vi "Impedance_Single_Meas.vi"(11 "Test Params Cluster":T1={"Test Freq. (Hz)"=1702.3933752476319, "Output Signal Amplitude\nVolts Pk"=0.1, "Sampling Time (s)"=0.01, "Sampling Rate (Hz)"=250000.0, "Output Channel"="Dev3/ao0", "Current Channel"="Dev3/ai1", "Voltage Channel"="Dev3/ai0", "Trigger Channel"="/Dev3/ao/StartTrigger", "Number of runs"=5}) -> (0 "Current Complex":cdb=0.1092230559688666-0.017870132117080606i, 1 "Voltage Complex":cdb=-0.17452167799153867-1.07754869267134i, 2 "Time domain Current":waveform(dbl)(graph)={"t0"=timestamp(3724535126.9386544 s since 1904-01-01), "dt"=3.999999999999989e-06, "Y"=array[2500 elements], "attributes"=variant("NI_ChannelName"=variant(string "Dev3/ai1"), "NI_UnitDescription"=variant(string "Volts"))}, 3 "Time domain Voltage":waveform(dbl)(graph)={"t0"=timestamp(3724535127.000671 s since 1904-01-01), "dt"=3.999999999999989e-06, "Y"=array[2500 elements], "attributes"=variant("NI_ChannelName"=variant(string "Dev3/ai0"), "NI_UnitDescription"=variant(string "Volts"))})   [LabVIEW 2022 SP3]
uses:
  <vilib>/DAQmx/write.llb/DAQmx Write (Analog Wfm 1Chan NSamp).vi
  <vilib>/DAQmx/read.llb/DAQmx Read (Analog 1D Wfm NChan NSamp).vi
  <vilib>/DAQmx/create/channels.llb/DAQmx Create Channel (AI-Voltage-Basic).vi
  <vilib>/DAQmx/create/channels.llb/DAQmx Create Channel (AO-Voltage-Basic).vi
  <vilib>/DAQmx/configure/timing.llb/DAQmx Timing (Sample Clock).vi
  <vilib>/DAQmx/miscellaneous.llb/DAQmx Fill In Error Info.vi
  <vilib>/DAQmx/configure/trigger.llb/DAQmx Start Trigger (Digital Edge).vi
  <vilib>/measure/matone.llb/Extract Single Tone Information 1 Chan.vi
  <vilib>/measure/NI_MABase.lvlib
  <vilib>/measure/NI_MAPro.lvlib
panel:
  out "Updated Cluster":T1
  out "Test Freq. (Hz)":dbl=1702.3933752476319
  out "Mag Current":dbl=0.1106752798824565
  in  "Use LabView\nSignal Detect":bool=TRUE
  out "detected phase (Rad)":dbl=4.551821517545998
  out "detected amplitude":dbl=1.0915901250774929 format="%.2p"
  in  "search (+/- % of Fsampl.)":dbl
  in  "advanced search":T2={"approx freq. (optional)"=-1.0, "search (+/- % of Fsampl.)"=5.0} {"search (+/- % of Fsampl.)" format="%0.2p"; "approx freq. (optional)" format="%0.2p"}
  out "Detected Time domain Current 2":waveform(dbl)(graph)={"t0"=timestamp(2.12 s since 1904-01-01), "dt"=4e-06, "Y"=array[2500 elements]}
  out "Detected Time domain Voltage 2":waveform(dbl)(graph)={"t0"=timestamp(2.13 s since 1904-01-01), "dt"=4e-06, "Y"=array[2500 elements]}
  out "detected frequency 2":dbl=1700.0000000000045 format="%.2p"
  out "detected frequency":dbl=1700.0000000000045 format="%.2p"
  out "Current phase (deg)":dbl=-0.16217447631966198 format="%.2p"
  out "Voltage phase (deg)":dbl=260.8001620522193 format="%.2p"
  in  "CurentRangeMax":dbl=5.0 format="%0.2f"
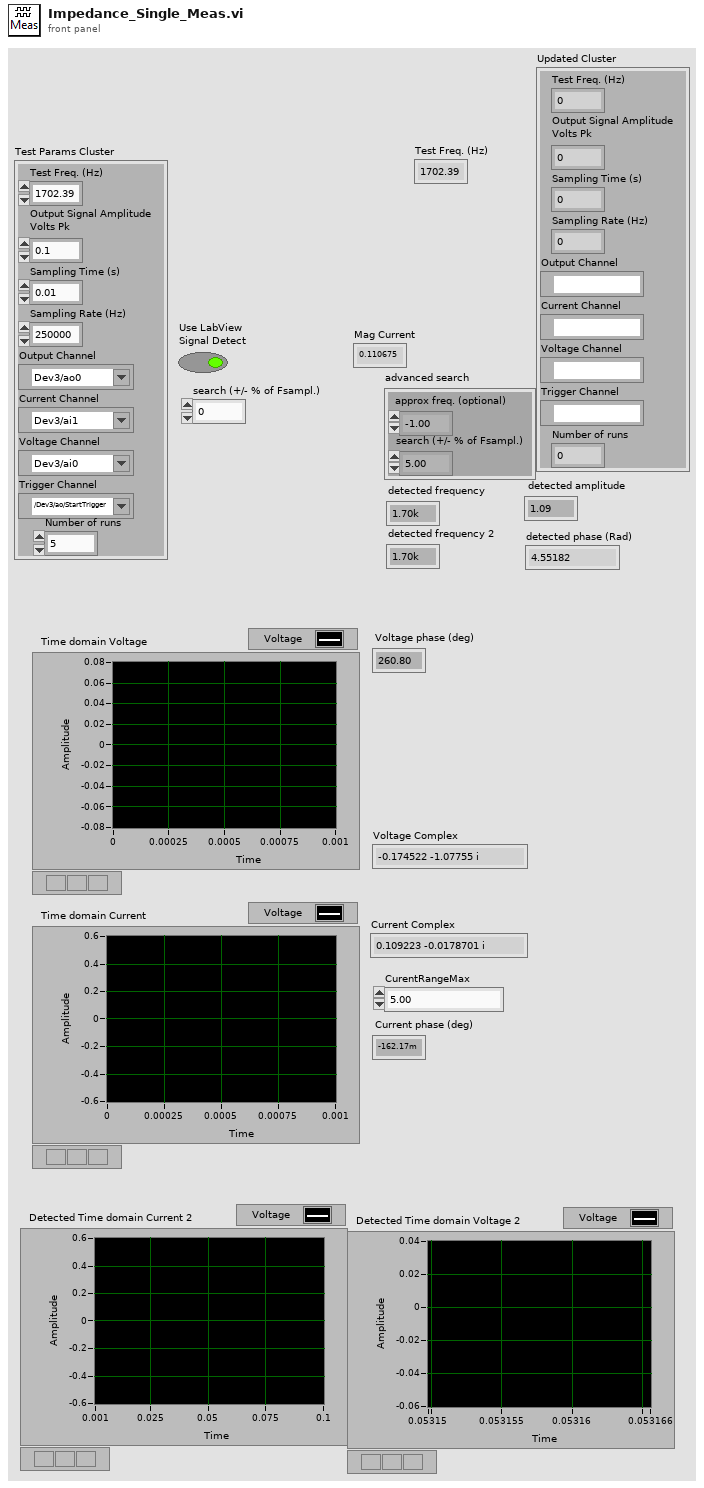
[diagram p1: front panel]
types:
  T1 = cluster{"Test Freq. (Hz)":dbl, "Output Signal Amplitude\nVolts Pk":dbl, "Sampling Time (s)":dbl, "Sampling Rate (Hz)":dbl, "Output Channel":tag, "Current Channel":tag, "Voltage Channel":tag, "Trigger Channel":tag, "Number of runs":i32}
  T2 = cluster{"approx freq. (optional)":dbl, "search (+/- % of Fsampl.)":dbl}
  T3 = enum32{"none", "input signal", "detected signal", "residual signal"}
  T4 = cluster{"exported time signal":waveform(dbl), "exported spectrum (dB)":cluster{"f0":dbl, "df":dbl, "dB Spectrum (Hann)":dbl[]}}
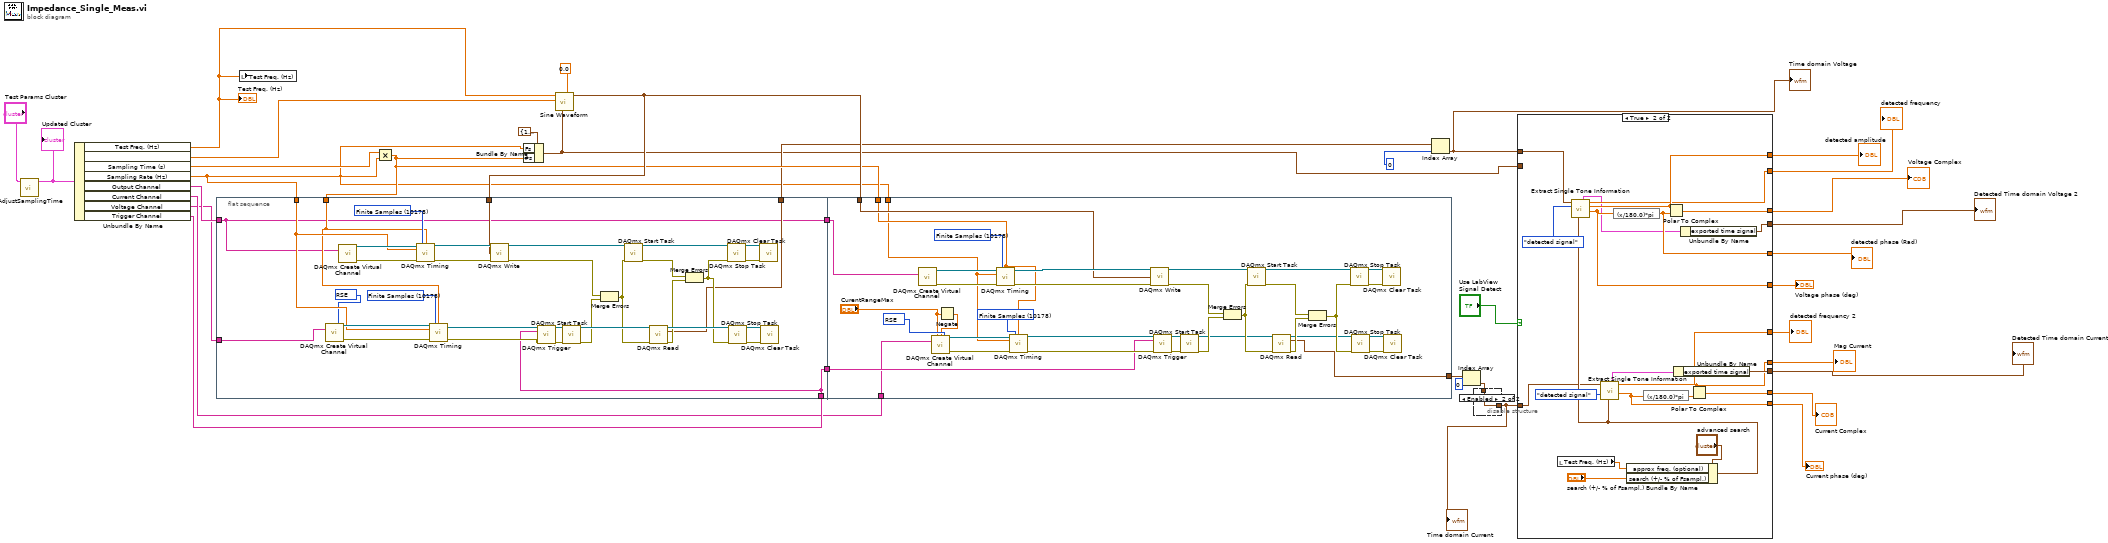
[diagram p0: block diagram]
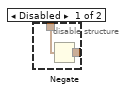
[diagram p2: hidden frame]
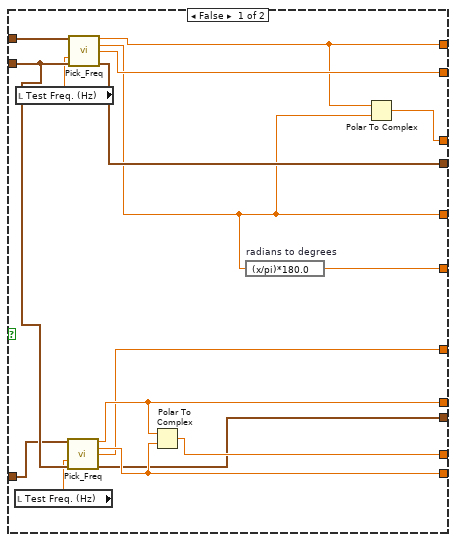
[diagram p3: hidden frame]
diagram:
  n1 = call "AdjustSamplingTime.vi"("Test Params Cluster"="Test Params Cluster") -> ("output cluster"=w2:T1)  [unwired: 10 in]
  "Updated Cluster" <- w2
  n2 = Unbundle By Name(w2) -> ("Test Freq. (Hz)"=w10:dbl, "Output Signal Amplitude\nVolts Pk"=w9:dbl, "Sampling Time (s)"=w8:dbl, "Sampling Rate (Hz)"=w7:dbl, "Output Channel"=w5:tag, "Current Channel"=w4:tag, "Voltage Channel"=w3:tag, "Trigger Channel"=w6:tag)
  "Test Freq. (Hz)" <- w10
  n3 = flat-sequence {
    tunnel: w7 -> [w48]
    tunnel: w32 -> [w47]
    tunnel: w33 -> [w46]
    tunnel: [w41] -> w29
    tunnel: [w40] -> w34
    tunnel: [w38] -> w22
    tunnel: w5 -> [w40]
    tunnel: w3 -> [w39]
    tunnel: w6 -> [w38]
    tunnel: w34 -> [w79]
    tunnel: [w78] -> w26
    tunnel: w33 -> [w77]
    tunnel: w32 -> [w76]
    tunnel: w7 -> [w75]
    tunnel: w22 -> [w72]
    tunnel: w4 -> [w71]
    frame #0 {
      w37 = 10083 items=["Default"=-1, "RSE"=10083, "NRSE"=10078, "Differential"=10106, "Pseudodifferential"=12529] ("input terminal configuration")
      w60 = 10178 items=["Finite Samples"=10178, "Continuous Samples"=10123, "Hardware Timed Single Point"=12522] ("sample mode")
      w63 = 10178 items=["Finite Samples"=10178, "Continuous Samples"=10123, "Hardware Timed Single Point"=12522] ("sample mode")
      n4 = call-poly <vilib>:"DAQmx Create Virtual Channel.vi"("input terminal configuration"=w37, "physical channels"=w39) -> ("task out"=w61:refnum<k21>, "error out"=w62:errorcluster)  [unwired: 12 in]
      n5 = call-poly <vilib>:"DAQmx Create Virtual Channel.vi"("physical channels"=w40) -> ("task out"=w70:refnum<k21>, "error out"=w66:errorcluster)  [unwired: 13 in]
      n6 = call-poly <vilib>:"DAQmx Timing.vi"("task/channels in"=w70, "sample mode"=w63, "samples per channel"=w47, "rate"=w48, "error in"=w66) -> ("task out"=w69:refnum<k21>, "error out"=w67:errorcluster)  [unwired: 9 in]
      n7 = call-poly <vilib>:"DAQmx Timing.vi"("task/channels in"=w61, "sample mode"=w60, "samples per channel"=w47, "rate"=w48, "error in"=w62) -> ("task out"=w59:refnum<k21>, "error out"=w58:errorcluster)  [unwired: 9 in]
      n8 = call-poly <vilib>:"DAQmx Write.vi"("task/channels in"=w69, "data"=w46, "error in"=w67) -> ("task out"=w68:refnum<k21>, "error out"=w50:errorcluster)  [unwired: 10 in, 1 out]
      n9 = call-poly <vilib>:"DAQmx Trigger.vi"("task/channels in"=w59, "source"=w38, "error in"=w58) -> ("task out"=w56:refnum<k21>, "error out"=w57:errorcluster)  [unwired: 11 in]
      n10 = call <vilib>:"DAQmx Start Task.vi"("task/channels in"=w56, "error in"=w57) -> ("task out"=w55:refnum<k21>, "error out"=w51:errorcluster)  [unwired: 12 in]
      n11 = Merge Errors(w50, w51) -> (w49:errorcluster)
      n12 = call <vilib>:"DAQmx Start Task.vi"("task/channels in"=w68, "error in"=w49) -> ("task out"=w65:refnum<k21>, "error out"=w43:errorcluster)  [unwired: 12 in]
      n13 = call-poly <vilib>:"DAQmx Read.vi"("task/channels in"=w55, "error in"=w49) -> ("task out"=w52:refnum<k21>, "data"=w41:waveform(dbl)[], "error out"=w44:errorcluster)  [unwired: 11 in]
      n14 = Merge Errors(w43, w44) -> (w42:errorcluster)
      n15 = call <vilib>:"DAQmx Stop Task.vi"("task/channels in"=w65, "error in"=w42) -> ("task out"=w64:refnum<k21>, "error out"=w45:errorcluster)  [unwired: 12 in]
      n16 = call <vilib>:"DAQmx Stop Task.vi"("task/channels in"=w52, "error in"=w42) -> ("task out"=w53:refnum<k21>, "error out"=w54:errorcluster)  [unwired: 12 in]
      n17 = call <vilib>:"DAQmx Clear Task.vi"("task in"=w64, "error in"=w45) -> ()  [unwired: 13 in, 1 out]
      n18 = call <vilib>:"DAQmx Clear Task.vi"("task in"=w53, "error in"=w54) -> ()  [unwired: 13 in, 1 out]
    }
    frame #1 {
      w102 = 10083 items=["Default"=-1, "RSE"=10083, "NRSE"=10078, "Differential"=10106, "Pseudodifferential"=12529] ("input terminal configuration")
      w90 = 10178 items=["Finite Samples"=10178, "Continuous Samples"=10123, "Hardware Timed Single Point"=12522] ("sample mode")
      w87 = 10178 items=["Finite Samples"=10178, "Continuous Samples"=10123, "Hardware Timed Single Point"=12522] ("sample mode")
      n19 = call-poly <vilib>:"DAQmx Create Virtual Channel.vi"("physical channels"=w79) -> ("task out"=w80:refnum<k21>, "error out"=w84:errorcluster)  [unwired: 13 in]
      n20 = Negate(x="CurentRangeMax") -> (-x=w73:dbl)
      n21 = call-poly <vilib>:"DAQmx Create Virtual Channel.vi"("maximum value"="CurentRangeMax", "minimum value"=w73, "input terminal configuration"=w102, "physical channels"=w71) -> ("task out"=w89:refnum<k21>, "error out"=w88:errorcluster)  [unwired: 10 in]
      n22 = call-poly <vilib>:"DAQmx Timing.vi"("task/channels in"=w80, "sample mode"=w87, "samples per channel"=w76, "rate"=w75, "error in"=w84) -> ("task out"=w81:refnum<k21>, "error out"=w83:errorcluster)  [unwired: 9 in]
      n23 = call-poly <vilib>:"DAQmx Timing.vi"("task/channels in"=w89, "sample mode"=w90, "samples per channel"=w76, "rate"=w75, "error in"=w88) -> ("task out"=w91:refnum<k21>, "error out"=w92:errorcluster)  [unwired: 9 in]
      n24 = call-poly <vilib>:"DAQmx Write.vi"("task/channels in"=w81, "data"=w77, "error in"=w83) -> ("task out"=w82:refnum<k21>, "error out"=w100:errorcluster)  [unwired: 10 in, 1 out]
      n25 = call-poly <vilib>:"DAQmx Trigger.vi"("task/channels in"=w91, "source"=w72, "error in"=w92) -> ("task out"=w94:refnum<k21>, "error out"=w93:errorcluster)  [unwired: 11 in]
      n26 = call <vilib>:"DAQmx Start Task.vi"("task/channels in"=w94, "error in"=w93) -> ("task out"=w95:refnum<k21>, "error out"=w99:errorcluster)  [unwired: 12 in]
      n27 = Merge Errors(w100, w99) -> (w101:errorcluster)
      n28 = call <vilib>:"DAQmx Start Task.vi"("task/channels in"=w82, "error in"=w101) -> ("task out"=w85:refnum<k21>, "error out"=w105:errorcluster)  [unwired: 12 in]
      n29 = call-poly <vilib>:"DAQmx Read.vi"("task/channels in"=w95, "error in"=w101) -> ("task out"=w98:refnum<k21>, "data"=w78:waveform(dbl)[], "error out"=w104:errorcluster)  [unwired: 11 in]
      n30 = Merge Errors(w105, w104) -> (w106:errorcluster)
      n31 = call <vilib>:"DAQmx Stop Task.vi"("task/channels in"=w85, "error in"=w106) -> ("task out"=w86:refnum<k21>, "error out"=w103:errorcluster)  [unwired: 12 in]
      n32 = call <vilib>:"DAQmx Stop Task.vi"("task/channels in"=w98, "error in"=w106) -> ("task out"=w97:refnum<k21>, "error out"=w96:errorcluster)  [unwired: 12 in]
      n33 = call <vilib>:"DAQmx Clear Task.vi"("task in"=w86, "error in"=w103) -> ()  [unwired: 13 in, 1 out]
      n34 = call <vilib>:"DAQmx Clear Task.vi"("task in"=w97, "error in"=w96) -> ()  [unwired: 13 in, 1 out]
    }
  }
  n35 = local write "Test Freq. (Hz)"(w10) -> ()
  n36 = Multiply(x=w8, y=w7) -> (x*y=w32:dbl)
  n37 = Bundle By Name(cluster=cluster{"Fs":dbl, "#s":dbl} {"Fs"=1000.0, "#s"=1000.0} ("sampling info"), "Fs"=w7, "#s"=w32) -> (w12:cluster{"Fs":dbl, "#s":dbl})
  n38 = call <vilib>:"Sine Waveform.vi"("offset"=0.0, "sampling info"=w12, "amplitude"=w9, "frequency"=w10) -> ("signal out"=w33:waveform(dbl))  [unwired: 6 in, 1 out]
  n39 = Index Array(array=w29, index=0) -> (element=w21:waveform(dbl))
  "Time domain Voltage" <- w21
  n40 = Index Array(array=w26, index=0) -> (element=w24:waveform(dbl))
  n41 = disable-structure shown="Enabled" {
    disable-tunnel: w24 -> [w108 w109]
    disable-tunnel: [w107 w109] -> w11
    frame Disabled {
      n42 = Negate(x=w108) -> (-x=w107:waveform(dbl))
    }
    frame Enabled {
    }
  }
  "Time domain Current" <- w11
  n43 = case shown="True" "Use LabView\nSignal Detect" {
    tunnel: [w115 w147] -> w31
    tunnel: [w114 w146] -> w30
    tunnel: [w116 w144] -> w25
    tunnel: [w124 w143] -> w23
    tunnel: w21 -> [w125 w137]
    tunnel: [w118 w136] -> w19
    tunnel: [w121 w135] -> w18
    tunnel: [w122 w134] -> w17
    tunnel: [w117 w133] -> w16
    tunnel: [w123 w128] -> w15
    tunnel: [w119 w130] -> w14
    tunnel: [w120 w129] -> w13
    tunnel: w12 -> [w113 _]
    tunnel: w11 -> [w112 w127]
    frame False {
      n44 = local read "Test Freq. (Hz)"() -> (w111:dbl)
      n45 = local read "Test Freq. (Hz)"() -> (w110:dbl)
      n46 = call "Pick_Freq.vi"("time signal"=w112, "RX frequency"=w111, "sampling info"=w113) -> ("Mag"=w123:dbl, "Phase"=w122:dbl, "actual freq"=w118:dbl, "signal out"=w119:waveform(dbl))  [unwired: 9 in]
      n47 = call "Pick_Freq.vi"("time signal"=w125, "RX frequency"=w110, "sampling info"=w113) -> ("Mag"=w115:dbl, "Phase"=w114:dbl, "actual freq"=w124:dbl, "signal out"=w120:waveform(dbl))  [unwired: 9 in]
      n48 = Polar To Complex(1:w122, 2:w123) -> (0:w121:cdb)
      n49 = expression code="(x/pi)*180.0" "radians to degrees"(w114) -> (w117:dbl)
      n50 = Polar To Complex(1:w114, 2:w115) -> (0:w116:cdb)
    }
    frame True {
      n51 = local read "Test Freq. (Hz)"() -> (w126:dbl)
      n52 = Bundle By Name(cluster="advanced search", "approx freq. (optional)"=w126, "search (+/- % of Fsampl.)"="search (+/- % of Fsampl.)") -> (w139:T2)
      n53 = call-poly <vilib>:"Extract Single Tone Information.vi"("advanced search"=w139, "export mode"=T3."detected signal", "time signal in"=w137) -> ("detected phase (deg)"=w133:dbl, "detected amplitude"=w147:dbl, "detected frequency"=w143:dbl, "exported signals"=w132:T4)  [unwired: 3 in, 2 out]
      n54 = call-poly <vilib>:"Extract Single Tone Information.vi"("advanced search"=w139, "export mode"=T3."detected signal", "time signal in"=w127) -> ("detected phase (deg)"=w134:dbl, "detected amplitude"=w128:dbl, "detected frequency"=w136:dbl, "exported signals"=w131:T4)  [unwired: 3 in, 2 out]
      n55 = expression code="(x/180.0)*pi" ("degrees to radians")(w133) -> (w146:dbl)
      n56 = expression code="(x/180.0)*pi" ("degrees to radians")(w134) -> (w145:dbl)
      n57 = Polar To Complex(1:w146, 2:w147) -> (0:w144:cdb)
      n58 = Unbundle By Name(w131) -> ("exported time signal"=w130:waveform(dbl))
      n59 = Unbundle By Name(w132) -> ("exported time signal"=w129:waveform(dbl))
      n60 = Polar To Complex(1:w145, 2:w128) -> (0:w135:cdb)
    }
  }
  "Voltage Complex" <- w25
  "detected frequency" <- w23
  "Detected Time domain Voltage 2" <- w13
  "Detected Time domain Current 2" <- w14
  "detected amplitude" <- w31
  "detected phase (Rad)" <- w30
  "detected frequency 2" <- w19
  "Current Complex" <- w18
  "Current phase (deg)" <- w17
  "Voltage phase (deg)" <- w16
  "Mag Current" <- w15
